vi "Handle Value Change.vi"(5 "VolatusAPI":refnum<class "VolatusAPI.lvclass">, 7 "CtlRef":refnum<vi>, 8 "error in (no error)":errorcluster, 9 "NewVal":variant, 10 "OldVal":variant, 11 "2WayValve in":refnum<class "2WayValveV.lvclass">) -> (0 "error out":errorcluster, 3 "2WayValve out":refnum<class "2WayValveV.lvclass">)   [LabVIEW 2020, in "VolatusGUIElements.lvlib" / "2WayValveV.lvclass"]
uses:
  2WayValveV.lvclass
  Volatus/VolatusAPI/VolatusAPI.lvclass
  2WayValveV.lvclass/2WayValveV.ctl
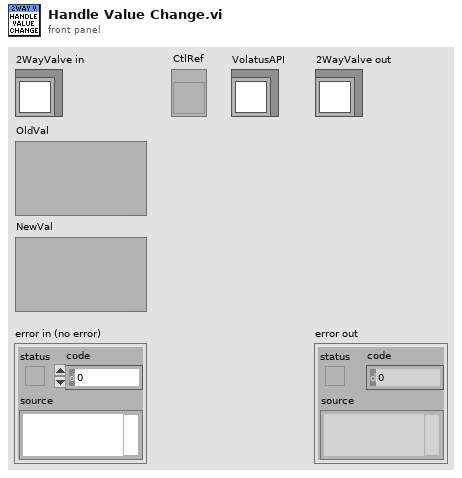
[diagram p1: front panel]
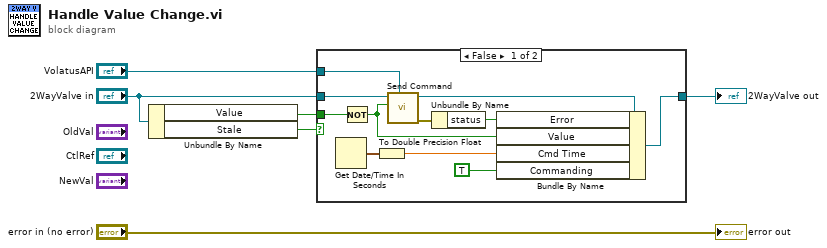
[diagram p0: block diagram]
diagram:
  n1 = Unbundle By Name("2WayValve in") -> ("Value"=w2:bool, "Stale"=w1:bool)
  n2 = case shown="False" w1 {
    tunnel: [w17 w18] -> w6
    tunnel: "VolatusAPI" -> [w15 _]
    tunnel: "2WayValve in" -> [w12 w18]
    tunnel: w2 -> [w11 _]
    frame False {
      n3 = Get Date/Time In Seconds() -> (seconds since 1Jan1904=w9:timestamp)
      n4 = Not(x=w11) -> (.not. x?=w10:bool)
      n5 = To Double Precision Float(number=w9) -> (double precision float=w8:dbl)
      n6 = call "Send Command.vi"("VolatusAPI"=w15, "Value"=w10, "2WayValve in"=w12) -> ("error out"=w14:errorcluster, "2WayValve out"=w16:refnum<class "2WayValveV.lvclass">)  [unwired: 7 in]
      n7 = Unbundle By Name(w14) -> ("status"=w13:bool)
      n8 = Bundle By Name(cluster=w16, "Error"=w13, "Value"=w10, "Cmd Time"=w8, "Commanding"=TRUE) -> (w17:refnum<class "2WayValveV.lvclass">)
    }
    frame True {
    }
  }
  "2WayValve out" <- w6
  "error out" <- "error in (no error)"
